vi "PmacCommError.vi"(0 "Input String":string) -> (1 "Error Bool (F)":bool, 2 "Output String":string, 3 "Error Number i32":i32=-1 min=-1 max=17, 4 "Error Message String (\"\")":string)   [LabVIEW 2020]
doc: "Parse Input String for PMAC ERR codes. This requires proper communication I-Variable configuration - see the PMACView manual. If an ERR code is found it is decoded and a modal dialog is displayed telling you the command that caused the error, a description of the error, and possible remedies. The user can decide to Abort execution of the application VI or ignore the error and Continue. With or without errors Output String is a copy of Input String after parsing.\n\nIf an error is found Error Bool is TRUE. Error Number and Error Message contain the error code and text description of the error. If no error is found Error Bool is FALSE. Error Number = -1 and Error Message is \"No Error\""
uses:
  PmacCommGlobal.vi
panel:
  in  "Error Message Table Private":string[](array[string])=["ERR:\nUnknown Error Source", "ERR001:\nCommand not allowed during program execution.\n\nSolution:\nHalt program execution before issuing command.\n", "ERR 002:\nPassword Error.\n\nSolution\nEnter proper password.", "ERR003:\nData error or unrecognized command.\n\nSolution:\nCorrect syntax of command.", "ERR004:\nIllegal character - bad value (>127 ASCII) or serial parity/framing error.\n\nSolution:\nCorrect character and/or check for noise on the serial cable.", "ERR005:\nCommand not allowed unless buffer is open.\n\nSolution:\nOpen buffer first.", "ERR006:\nNo room in buffer for command.\n\nSolution:\nAllow more room for buffer.  DELETE or CLEAR other buffers.", "ERR007:\nBuffer already in use.\n\nSolution:\nCLOSE currently open buffer first.", "ERR008:\nReserved for future use.", "ERR009:\nProgram structural error (e.g. ENDIF without IF)\n\nSolution:\nCorrect structure of program.", "ERR010:\nBoth overtravel limits set for a motor in the C.S.\n\nSolution:\nCorrect of disable limits.", "ERR011:\nPrevious move not completed.\n\nSolution:\nABORT it or allow it to complete.", "ERR012:\nA motor in the coordinate system is open loop.\n\nSolution:\nClose the loop on the motor.", "ERR013:\nA motor in the coordinate system is not activated.\n\nSolution:\nSet Ix00 to 1 or remove motor from the C.S..", "ERR014:\nNo motors in the coordinate system.\n\nSolution:\nDefine at least one motor in the C.S..", "ERR015:\nNot pointing to valid program buffer.\n\nSolution:\nUse B command first, or clear out scrambled buffers.", "ERR016:\nRunning improperly structured program (e.g.) missing ENDWHILE.\n\nSolution:\nCorrect structure of program.", "ERR017:\nMotor(s) in C.S. not at halted position to restart after / or \\ command.\n\nSolution:\nMove motors back to halted position with J=."]
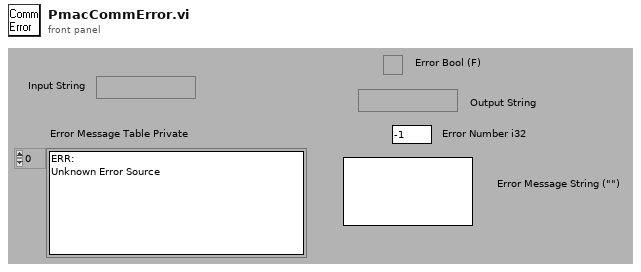
[diagram p1: front panel]
types:
  T1 = cluster{"Command String":string, "Response String":string, "Communication Log String":string, "Num Commands i32":i32, "Buffer Log Bool (F)":bool}
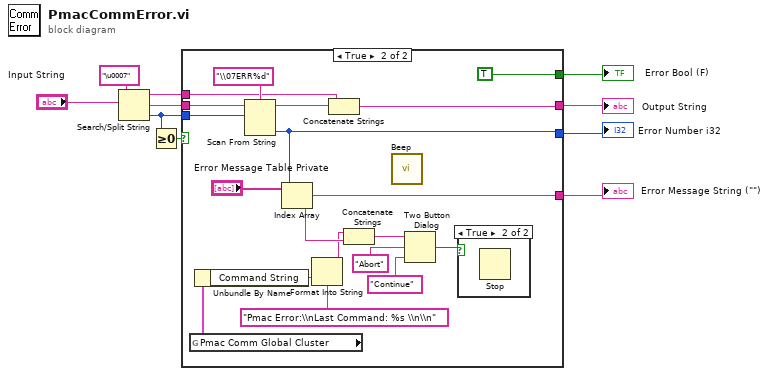
[diagram p0: block diagram]
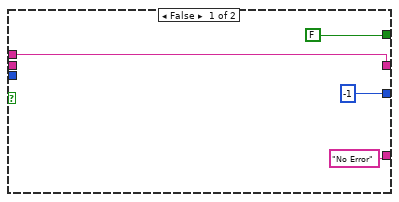
[diagram p2: hidden frame]
diagram:
  n1 = Search/Split String(string="Input String", search string/char (-)="\u0007") -> (substring before match=w7:string, match + rest of string=w8:string, offset of match=w6:i32)  [unwired: 1 out]
  n2 = Greater Or Equal To 0?(x=w6) -> (x >= 0?=w5:bool)
  n3 = case shown="True" w5 {
    tunnel: w8 -> [_ w31]
    tunnel: [w14 w24] -> w2
    tunnel: w7 -> [w14 w25]
    tunnel: [-1 w28] -> w3
    tunnel: w6 -> [_ w30]
    tunnel: ["No Error" w27] -> w4
    tunnel: [FALSE TRUE] -> w1
    frame False {
    }
    frame True {
      n4 = global read "PmacCommGlobal.vi" "Pmac Comm Global Cluster"() -> (w19:T1)
      n5 = Unbundle By Name(w19) -> ("Command String"=w20:string)
      n6 = Scan From String(format string="\\07ERR%d", input string=w31, initial scan location=w30) -> (remaining string=w26:string, output 1=w28:i32)  [unwired: 1 in, 3 out]
      n7 = Index Array(array="Error Message Table Private", index=w28) -> (element=w27:string)
      n8 = Format Into String(format string="Pmac Error:\\nLast Command: %s \\n\\n", w20) -> (resulting string=w17:string)  [unwired: 2 in, 1 out]
      n9 = Concatenate Strings(w25, w26) -> (w24:string)
      n10 = Concatenate Strings(w17, w27) -> (w16:string)
      n11 = call <vilib>:"Beep.vi"() -> ()  [unwired: 3 in, 9 out]
      n12 = Two Button Dialog(message=w16, 1:"Continue", 2:"Abort") -> (T button?=w15:bool)
      n13 = case shown="True" w15 {
        frame False {
        }
        frame True {
          n14 = Stop() -> ()  [unwired: 1 out]
        }
      }
    }
  }
  "Output String" <- w2
  "Error Number i32" <- w3
  "Error Message String (\"\")" <- w4
  "Error Bool (F)" <- w1
